vi "(SubVI) Split string.vi"(1 "text":string) -> (0 "text array":string[](array[string]))   [LabVIEW 2022 SP3]
uses:
  <vilib>/Utility/error.llb/Trim Whitespace One-Sided.vi
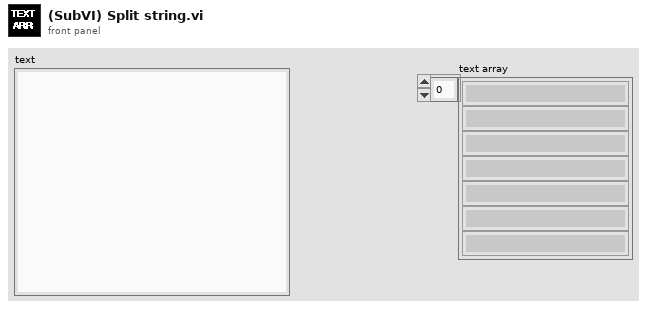
[diagram p1: front panel]
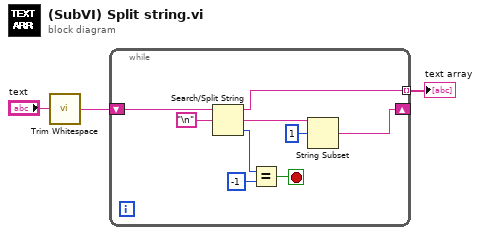
[diagram p0: block diagram]
diagram:
  n1 = call <vilib>:"Trim Whitespace.vi"("string"="text") -> ("trimmed string"=w3:string)  [unwired: 1 in]
  n2 = while {
    shift-right: [w5] -> _
    shift-left: w3 -> [w12]
    tunnel: [w4] -> w1 mode=indexing
    stop <- w8 stop-if-true
    n3 = Search/Split String(string=w12, search string/char (-)="\n") -> (substring before match=w4:string, match + rest of string=w6:string, offset of match=w10:i32)  [unwired: 1 in]
    n4 = Equal?(x=w10, y=-1) -> (x = y?=w8:bool)
    n5 = String Subset(string=w6, offset (0)=1) -> (substring=w5:string)  [unwired: 1 in]
  }
  "text array" <- w1
